vi "Launch Command.vi"(8 "error in (no error)":errorcluster, 9 "Command Name In":string, 10 "Command In":refnum<class "Command.lvclass">, 11 "Command Processor in":refnum<class "Command Processor.lvclass">) -> (0 "error out":errorcluster, 1 "Command Name Out":string, 2 "Command Out":refnum<class "Command.lvclass">, 3 "Command Processor out":refnum<class "Command Processor.lvclass">)   [LabVIEW 2013, in "Robot Actors.lvlib" / "Command Processor.lvlib" / "Command Processor.lvclass"]
uses:
  Command Processor.lvclass
  Command/Command Class/Command.lvclass
  <vilib>/ActorFramework/Actor/Actor.lvclass/Actor.ctl
  <vilib>/ActorFramework/Message Enqueuer/Message Enqueuer.lvclass/Message Enqueuer.ctl
  <vilib>/ActorFramework/Message Enqueuer/Init from Existing Queue.vi
  <vilib>/ActorFramework/Message Enqueuer/Message Enqueuer.lvclass
  <vilib>/ActorFramework/Actor/Actor.lvclass
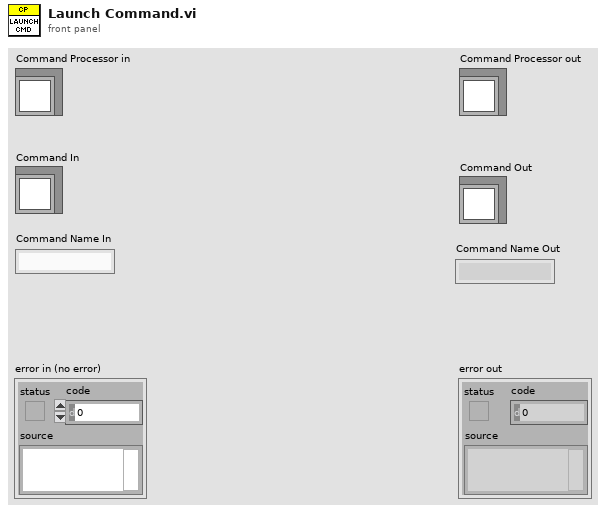
[diagram p1: front panel]
types:
  T1 = typedef "Robot Actors.lvlib/Command Processor.lvlib/Command Processor.lvclass/Command Processor Status.ctl" = cluster{"Next Command ID":dbl, "Current Command Status":T2, "Previous Command Status ":T2, "Command Processor State":T4, "Last Status Update":timestamp}
  T2 = typedef "Robot Actors.lvlib/Command.lvlib/Command.lvclass/Command Status.ctl" = cluster{"Command Name":string, "Command Start Time":timestamp, "Command End Time":timestamp, "Is Command Finished?":bool, "Command ID":dbl, "Command State":T3}
  T3 = typedef "Robot Actors.lvlib/Command.lvlib/Command.lvclass/Command States.ctl" = enum16{"Unknown", "Started", "Stopped", "Finished"}
  T4 = typedef "Robot Actors.lvlib/Command Processor.lvlib/Command Processor.lvclass/Command Processor States.ctl" = enum16{"Unknown", "No Command", "Running Command"}
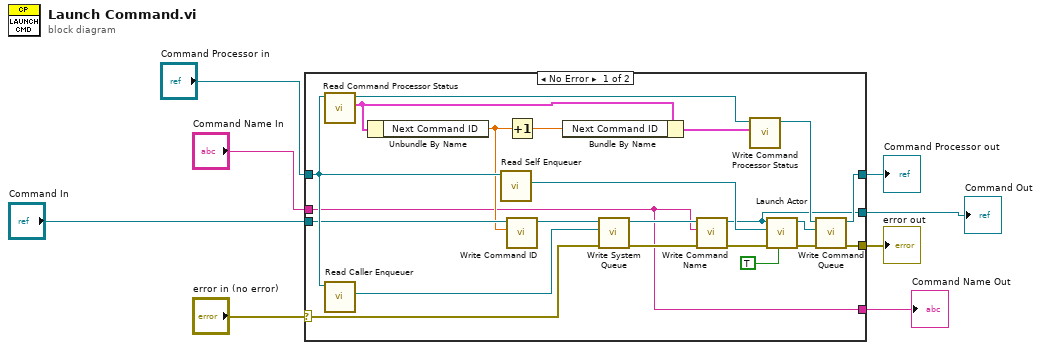
[diagram p0: block diagram]
diagram:
  n1 = case shown="No Error" "error in (no error)" {
    selector: "error in (no error)" -> [w23 w34]
    tunnel: [w21 w34] -> w7
    tunnel: [w22 w33] -> w5
    tunnel: "Command Processor in" -> [w19 w33]
    tunnel: "Command Name In" -> [w10 w32]
    tunnel: "Command In" -> [w15 w31]
    tunnel: [w10 w32] -> w2
    tunnel: [w9 w31] -> w1
    frame No Error {
      n2 = call-dynamic "Read Command Processor Status.vi"("Command Processor in"=w19) -> ("Command Processor Status"=w16:T1, "Command Processor out"=w17:refnum<class "Command Processor.lvclass">)  [unwired: 8 in, 1 out]
      n3 = call <vilib>:"Read Caller Enqueuer.vi"("Actor"=w19) -> ("Caller Enqueuer"=w24:refnum<class "Message Enqueuer.lvclass">)  [unwired: 10 in]
      n4 = Unbundle By Name(w16) -> ("Next Command ID"=w12:dbl)
      n5 = call <vilib>:"Read Self Enqueuer.vi"("Actor"=w19) -> ("Self Enqueuer"=w27:refnum<class "Message Enqueuer.lvclass">)  [unwired: 10 in]
      n6 = Increment(x=w12) -> (x+1=w11:dbl)
      n7 = call-dynamic "Write Command ID.vi"("Command ID"=w12, "Command in"=w15) -> ("Command out"=w14:refnum<class "Command.lvclass">)  [unwired: 8 in, 1 out]
      n8 = Bundle By Name(cluster=w16, "Next Command ID"=w11) -> (w13:T1)
      n9 = call-dynamic "Write System Queue.vi"("error in (no error)"=w23, "Actor Framework:Message Enqueuer"=w24, "Command in"=w14) -> ("error out"=w25:errorcluster, "Command out"=w26:refnum<class "Command.lvclass">)  [unwired: 7 in]
      n10 = call-dynamic "Write Command Name.vi"("error in (no error)"=w25, "Command Name"=w10, "Command in"=w26) -> ("error out"=w29:errorcluster, "Command out"=w9:refnum<class "Command.lvclass">)  [unwired: 7 in]
      n11 = call-dynamic "Write Command Processor Status.vi"("Command Processor Status"=w13, "Command Processor in"=w17) -> ("Command Processor out"=w18:refnum<class "Command Processor.lvclass">)  [unwired: 8 in, 1 out]
      n12 = call <vilib>:"Launch Actor.vi"("Open Actor Core front panel? (F)"=TRUE, "error in (no error)"=w29, "Actor-to-Caller Enqueuer"=w27, "Actor"=w9) -> ("error out"=w28:errorcluster, "Caller-To-Actor Enqueuer"=w30:refnum<class "Message Enqueuer.lvclass">)  [unwired: 6 in]
      n13 = call-dynamic "Write Command Queue.vi"("error in (no error)"=w28, "Actor Framework:Message Enqueuer"=w30, "Command Processor in"=w18) -> ("error out"=w21:errorcluster, "Command Processor out"=w22:refnum<class "Command Processor.lvclass">)  [unwired: 7 in]
    }
    frame Error {
    }
  }
  "error out" <- w7
  "Command Processor out" <- w5
  "Command Name Out" <- w2
  "Command Out" <- w1
